vi "Check Name.vi"(11 "XML Node Name":string) -> (0 "Error Out":errorcluster)   [LabVIEW 2019, in "Tree Map.lvlib"]
doc: "<b>Author:</b> Piotr Kruczkowski <PrimaryKey>\n<b>License:</b> NewBSD\n\nCopyright (c) 2019, National Instruments\nAll rights reserved.\n\nRedistribution and use in source and binary forms, with or without\nmodification, are permitted provided that the following conditions are met:\n1. Redistributions of source code must retain the above copyright\n notice, this list of conditions and the following disclaimer.\n2. Redistributions in binary form must reproduce the above copyright\n notice, this list of conditions and the following disclaimer in the\n documentation and/or other materials provided with the distribution.\n3. Neither the name of National Instruments nor the\n names of its contributors may be used to endorse or promote products\n derived from this software without specific prior written permission.\n\nTHIS SOFTWARE IS PROVIDED BY National Instruments ''AS IS'' AND ANY\nEXPRESS OR IMPLIED WARRANTIES, INCLUDING, BUT NOT LIMITED TO, THE IMPLIED\nWARRANTIES OF MERCHANTABILITY AND FITNESS FOR A PARTICULAR PURPOSE ARE\nDISCLAIMED. IN NO EVENT SHALL National Instruments BE LIABLE FOR ANY\nDIRECT, INDIRECT, INCIDENTAL, SPECIAL, EXEMPLARY, OR CONSEQUENTIAL DAMAGES\n(INCLUDING, BUT NOT LIMITED TO, PROCUREMENT OF SUBSTITUTE GOODS OR SERVICES;\nLOSS OF USE, DATA, OR PROFITS; OR BUSINESS INTERRUPTION) HOWEVER CAUSED AND\nON ANY THEORY OF LIABILITY, WHETHER IN CONTRACT, STRICT LIABILITY, OR TORT\n(INCLUDING NEGLIGENCE OR OTHERWISE) ARISING IN ANY WAY OUT OF THE USE OF THIS\nSOFTWARE, EVEN IF ADVISED OF THE POSSIBILITY OF SUCH DAMAGE."
uses:
  Tree Map.lvlib
panel:
  out "after substring":string
  out "before substring":string
  out "match substring":string
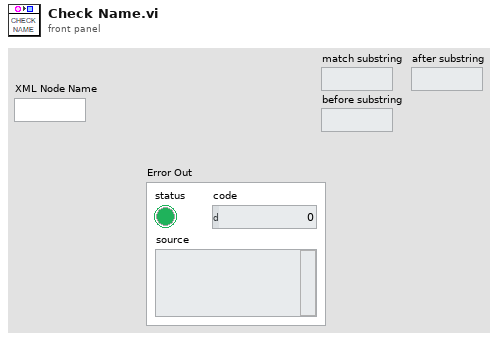
[diagram p1: front panel]
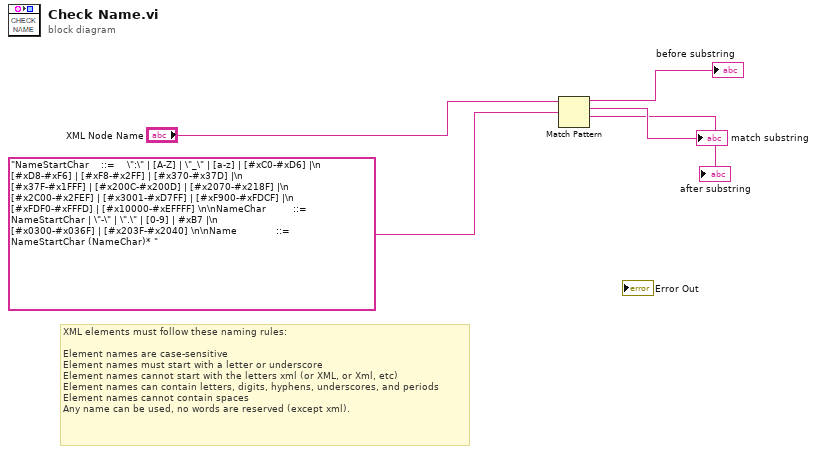
[diagram p0: block diagram]
diagram:
  # "XML elements must follow these naming rules:\n\nElement names are case-sensitive\nElement names must start with a letter or underscore\nElement names cannot start with the letters xml (or XML, or Xml, etc)\nElement names can contain letters, digits, hyphens, underscores, and periods\nElement names cannot contain spaces\nAny name can be used, no words are reserved (except xml)."
  n1 = Match Pattern(string="XML Node Name", regular expression="NameStartChar    ::=    \":\" | [A-Z] | \"_\" | [a-z] | [#xC0-#xD6] |\n                        [#xD8-#xF6] | [#xF8-#x2FF] | [#x370-#x37D] |\n                        [#x37F-#x1FFF] | [#x200C-#x200D] | [#x2070-#x218F] |\n                        [#x2C00-#x2FEF] | [#x3001-#xD7FF] | [#xF900-#xFDCF] |\n                        [#xFDF0-#xFFFD] | [#x10000-#xEFFFF] \n\nNameChar         ::=    NameStartChar | \"-\" | \".\" | [0-9] | #xB7 |\n                        [#x0300-#x036F] | [#x203F-#x2040] \n\nName             ::=    NameStartChar (NameChar)* ") -> (before substring=→"before substring":string, match substring=→"match substring":string, after substring=→"after substring":string)  [unwired: 1 in, 1 out]
